vi "_FPGA_Driver_LTC1667_3_v1.3.vi"(8 "Clk":bool, 10 "Data_in":fxp<+,14,14>) -> ()   [LabVIEW 2018]
uses:
  <vilib>/rvi/eio/common/nirviEmuTemplateMethod_errors.vi
  <vilib>/eio/EIONode/EIONode.xnode
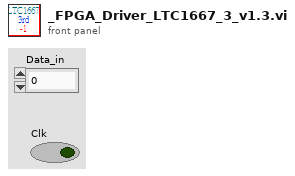
[diagram p1: front panel]
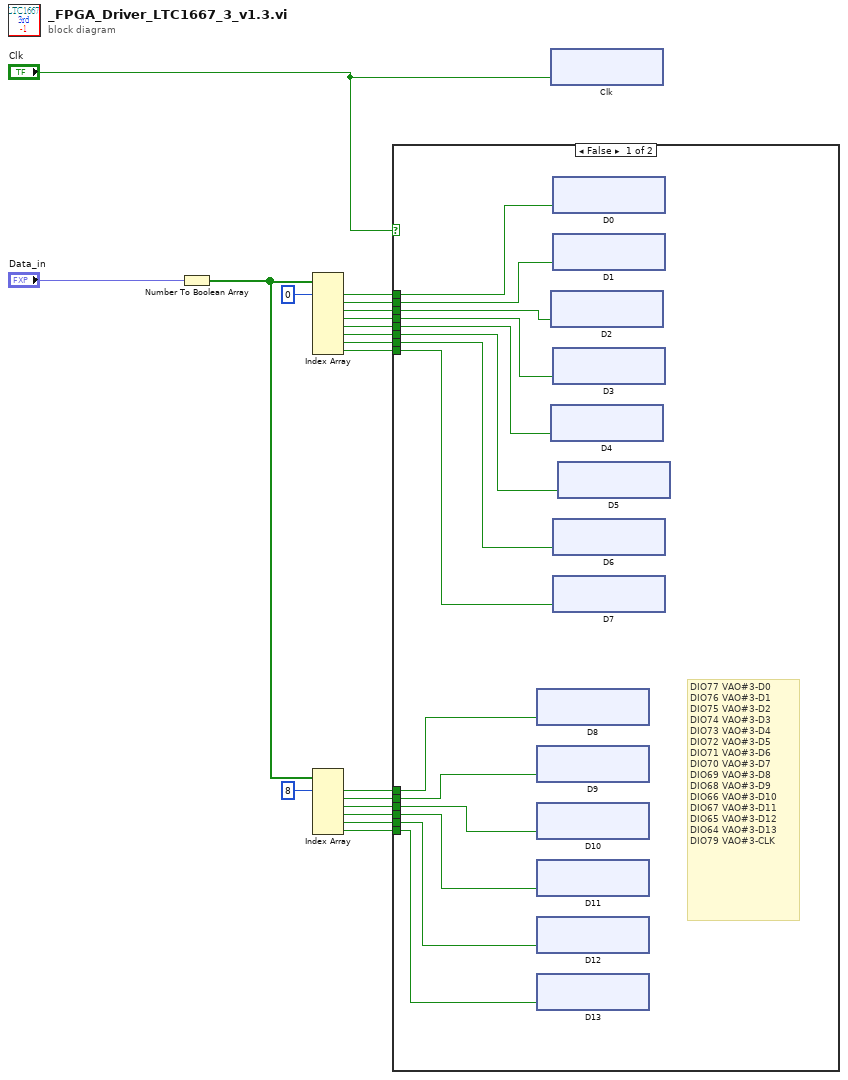
[diagram p0: block diagram]
diagram:
  n1 = Number To Boolean Array(number="Data_in") -> (Boolean array=w18:bool[])
  n2 = Index Array(array=w18, index #1=0 ("index")) -> (element #1=w16:bool, element #2=w15:bool, element #3=w14:bool, element #4=w13:bool, element #5=w12:bool, element #6=w11:bool, element #7=w10:bool, element #8=w9:bool)  [unwired: 7 in]
  n3 = Index Array(array=w18, index #1=8 ("index")) -> (element #1=w8:bool, element #2=w7:bool, element #3=w6:bool, element #4=w5:bool, element #5=w4:bool, element #6=w3:bool)  [unwired: 5 in]
  n4 = case shown="False" "Clk" {
    tunnel: w16 -> [w33 _]
    tunnel: w15 -> [w32 _]
    tunnel: w14 -> [w31 _]
    tunnel: w13 -> [w30 _]
    tunnel: w12 -> [w29 _]
    tunnel: w11 -> [w28 _]
    tunnel: w10 -> [w27 _]
    tunnel: w9 -> [w26 _]
    tunnel: w8 -> [w25 _]
    tunnel: w7 -> [w24 _]
    tunnel: w6 -> [w23 _]
    tunnel: w5 -> [w22 _]
    tunnel: w4 -> [w21 _]
    tunnel: w3 -> [w20 _]
    frame False {
      # "DIO77\tVAO#3-D0\nDIO76\tVAO#3-D1\nDIO75\tVAO#3-D2\nDIO74\tVAO#3-D3\nDIO73\tVAO#3-D4\nDIO72\tVAO#3-D5\nDIO71\tVAO#3-D6\nDIO70\tVAO#3-D7\nDIO69\tVAO#3-D8\nDIO68\tVAO#3-D9\nDIO66\tVAO#3-D10\nDIO67\tVAO#3-D11\nDIO65\tVAO#3-D12\nDIO64\tVAO#3-D13\nDIO79\tVAO#3-CLK"
      n5 = xnode "D8"("RMC/DIO69"=w25) -> ()  [unwired: 1 in, 1 out]
      n6 = xnode "D9"("RMC/DIO68"=w24) -> ()  [unwired: 1 in, 1 out]
      n7 = xnode "D10"("RMC/DIO66"=w23) -> ()  [unwired: 1 in, 1 out]
      n8 = xnode "D11"("RMC/DIO67"=w22) -> ()  [unwired: 1 in, 1 out]
      n9 = xnode "D12"("RMC/DIO65"=w21) -> ()  [unwired: 1 in, 1 out]
      n10 = xnode "D13"("RMC/DIO64"=w20) -> ()  [unwired: 1 in, 1 out]
      n11 = xnode "D2"("RMC/DIO75"=w31) -> ()  [unwired: 1 in, 1 out]
      n12 = xnode "D4"("RMC/DIO73"=w29) -> ()  [unwired: 1 in, 1 out]
      n13 = xnode "D0"("RMC/DIO77"=w33) -> ()  [unwired: 1 in, 1 out]
      n14 = xnode "D1"("RMC/DIO76"=w32) -> ()  [unwired: 1 in, 1 out]
      n15 = xnode "D3"("RMC/DIO74"=w30) -> ()  [unwired: 1 in, 1 out]
      n16 = xnode "D6"("RMC/DIO71"=w27) -> ()  [unwired: 1 in, 1 out]
      n17 = xnode "D7"("RMC/DIO70"=w26) -> ()  [unwired: 1 in, 1 out]
      n18 = xnode "D5"("RMC/DIO72"=w28) -> ()  [unwired: 1 in, 1 out]
    }
    frame True {
    }
  }
  n19 = xnode "Clk"("RMC/DIO79"="Clk") -> ()  [unwired: 1 in, 1 out]
